vi "Test Streams FG.vi"(9 "Remove":bool, 10 "Add":bool, 11 "Stream":refnum<class "WebsocketStream.lvclass">) -> (2 "Streams":refnum<class "WebsocketStream.lvclass">[](array[class]))   [LabVIEW 2020]
uses:
  Stream-Websocket/WebsocketStream/WebsocketStream.lvclass
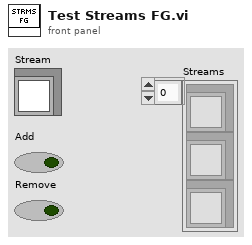
[diagram p1: front panel]
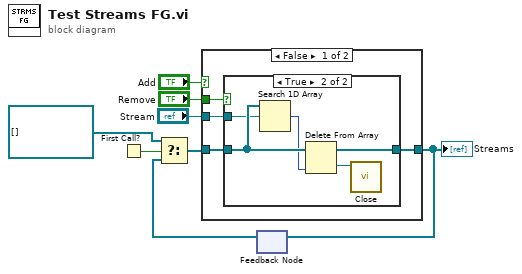
[diagram p0: block diagram]
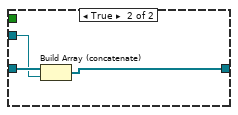
[diagram p3: hidden frame]
diagram:
  n1 = First Call?() -> (First Call?: T/F=w5:bool)
  n2 = feedback #1() -> (w4:refnum<class "WebsocketStream.lvclass">[])  [unwired: 1 in]
  n3 = Select(t=refnum<class "WebsocketStream.lvclass">[] [], s=w5, f=w4) -> (s? t:f=w2:refnum<class "WebsocketStream.lvclass">[])
  n4 = case shown="False" "Add" {
    tunnel: "Remove" -> [w12 _]
    tunnel: "Stream" -> [w9 w20]
    tunnel: w2 -> [w11 w21]
    tunnel: [w10 w19] -> w1
    frame False {
      n5 = case shown="True" w12 {
        tunnel: w11 -> [w13 w18]
        tunnel: [w13 w16] -> w10
        tunnel: w9 -> [_ w15]
        frame False {
        }
        frame True {
          n6 = Search 1D Array(1D array=w18, element=w15) -> (index of element=w17:i32)  [unwired: 1 in]
          n7 = Delete From Array(array=w18, index=w17) -> (deleted portion=w14:refnum<class "WebsocketStream.lvclass">, array with subset deleted=w16:refnum<class "WebsocketStream.lvclass">[])  [unwired: 1 in]
          n8 = call-dynamic "Close.vi"("WebsocketStream in"=w14) -> ()  [unwired: 9 in, 2 out]
        }
      }
    }
    frame True {
      n9 = Build Array (concatenate)(w21, w20) -> (w19:refnum<class "WebsocketStream.lvclass">[])
    }
  }
  "Streams" <- w1
  n10 = feedback-in #1(w1) -> ()
